vi "Current Target DAO.vi"(6 "Combined":bool, 7 "Use Offsets":bool caption="CartesianType", 8 "error in (no error)":errorcluster, 9 "Targets In":T1[](array[typedef]), 11 "DAO Actions":T3) -> (0 "error out":errorcluster, 1 "Targets  Out":T1[](array[typedef]))   [LabVIEW 2013]
uses:
  MixedMode/Messages/Target.ctl
  Data Access Objects/Metadata/LBCB Number.ctl
  Data Access Objects/Metadata/DAO Actions.ctl
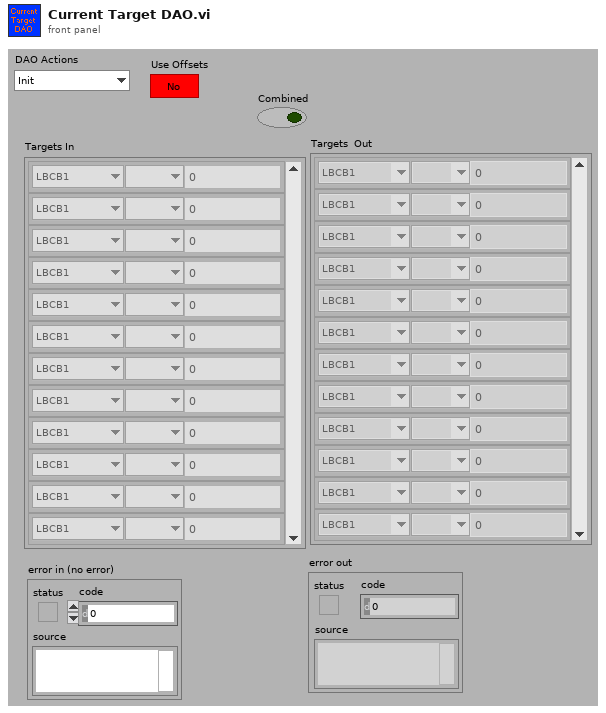
[diagram p1: front panel]
types:
  T1 = typedef "Target.ctl" = cluster{"LBCB Number":T2, "DOF Vectors":enum16{" ", "Dx", "Dy", "Dz", "Rx", "Ry", "Rz", "Fx", "Fy", "Fz", "Mx", "My", "Mz"}, "Amount":dbl}
  T2 = typedef "LBCB Number.ctl" = enum16{"LBCB1", "LBCB2"}
  T3 = typedef "DAO Actions.ctl" = enum16{"Init", "Get", "Set"}
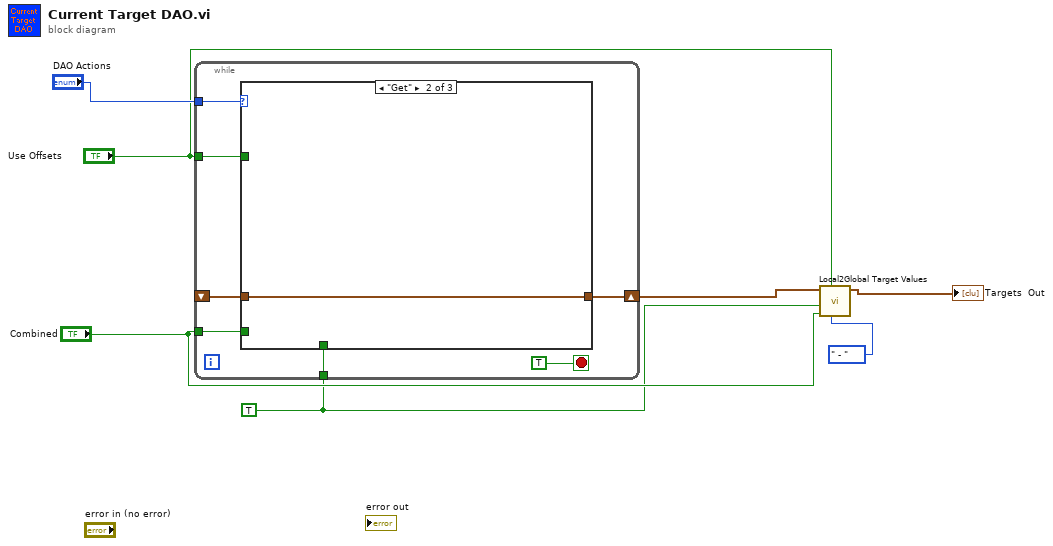
[diagram p0: block diagram]
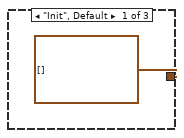
[diagram p2: hidden frame]
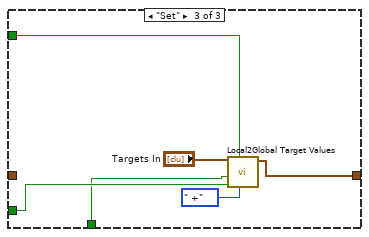
[diagram p3: hidden frame]
diagram:
  w1 = TRUE ("AreCommands")
  n1 = while {
    tunnel: "DAO Actions" -> [w13]
    tunnel: "Use Offsets" -> [w11]
    tunnel: "Combined" -> [w10]
    shift-right: [w12] -> w6
    shift-left: _ -> [w9]
    tunnel: w1 -> [w8]
    stop <- TRUE stop-if-true
    n2 = case shown="\"Get\"" w13 {
      tunnel: [T1[] [] ("Target  Outputs") w16 w21] -> w12
      tunnel: w11 -> [_ _ w20]
      tunnel: w10 -> [_ _ w19]
      tunnel: w9 -> [_ w16 _]
      tunnel: w8 -> [_ _ w17]
      frame "Init", Default {
      }
      frame "Get" {
      }
      frame "Set" {
        n3 = call "Local2Global Target Values.vi"("Direction"=enum16{" +", " - "}." +", "Use Offsets"=w20, "Combined"=w19, "AreCommands"=w17, "Target  Inputs"="Targets In") -> ("Target  Outputs"=w21:T1[])  [unwired: 6 in]
      }
    }
  }
  n4 = call "Local2Global Target Values.vi"("Direction"=enum16{" +", " - "}." - ", "Use Offsets"="Use Offsets", "Combined"="Combined", "AreCommands"=w1, "Target  Inputs"=w6) -> ("Target  Outputs"=→"Targets  Out":T1[])  [unwired: 6 in]
